vi "NVH_TEST.vi"(10 "振动2NHV-FFT":refnum<vi>, 11 "振动1NVH-FFT":refnum<vi>) -> ()   [LabVIEW 2020]
uses:
  Global_Variable/Global.vi
panel:
  out "error out":errorcluster caption="错误输出"
  in  "error in":errorcluster caption="错误输入"
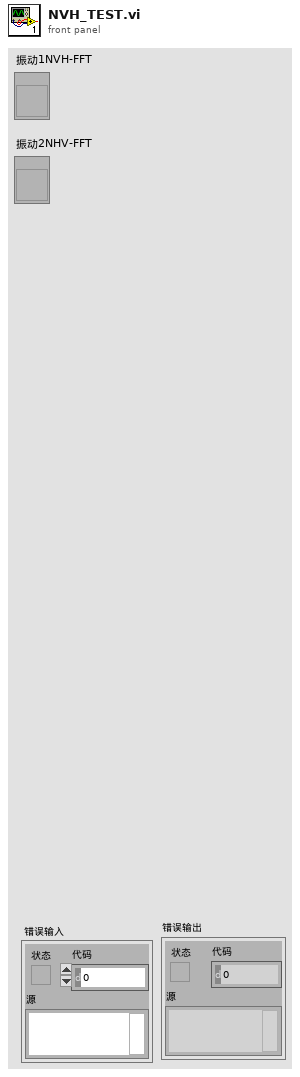
[diagram p1: front panel]
types:
  T1 = typedef "svc_Spectrum Info.ctl" = cluster{"channel name":string, "description":string, "x-axis units":T2, "spectral info":cluster{"spectrum type":T3, "linear/dB":enum16{"linear", "dB"}, "window":u16, "window size":i32, "FFT size":i32}, "engineering units":T4, "custom label":string, "dB reference [EU]":dbl, "peak units":enum16{"rms", "peak", "peak-peak"}, "weighting filter":T5, "spectral density?":bool, "unit label":string, "spectrum skewed?":bool, "complimentary spectrum units":T6}
  T2 = typedef "svc_X-Axis Units.ctl" = u16
  T3 = typedef "svc_Spectrum Type.ctl" = enum16{"FFT Spectrum [complex]", "Amplitude [Magnitude]", "Power [Magnitude^2]", "Cross Spectrum [complex]", "Frequency Response [Complex]"}
  T4 = typedef "svc_Engineering Units Text Ring.ctl" = u16
  T5 = typedef "svc_Weighting Filter Text Ring.ctl" = u16
  T6 = typedef "svc_Complimentary Spectrum Units.ctl" = enum16{"none", "radians", "degrees", "cycles", "imaginary"}
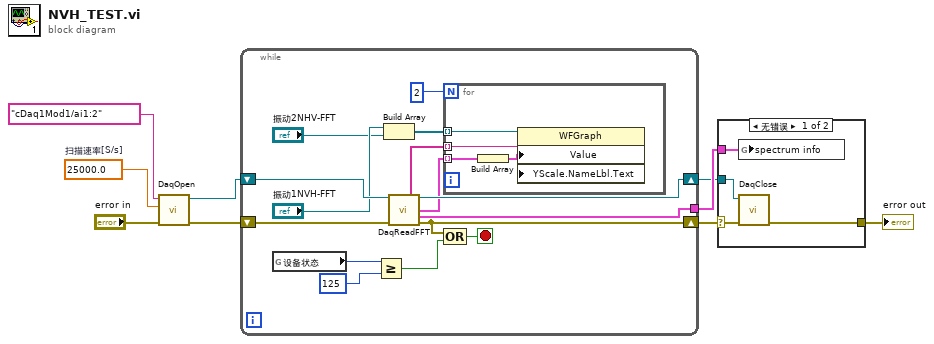
[diagram p0: block diagram]
diagram:
  w1 = 25000.0  # 扫描速率[S/s]
  n1 = call "DaqOpen.vi"("error in"="error in", "扫描速率[S/s]"=w1, "通道输入"=tag "cDaq1Mod1/ai1:2" ("DAQmx物理通道")) -> ("error out"=w9:errorcluster, "task out"=w3:refnum<k21>)  [unwired: 7 in]
  n2 = while {
    shift-right: [w23] -> w4
    shift-left: w3 -> [w24]
    shift-right: [w22] -> w5
    shift-left: w9 -> [w19]
    tunnel: [w20] -> w7
    stop <- w21 stop-if-true
    n3 = global read "Global.vi" "设备状态"() -> (w11:i16)
    n4 = Greater Or Equal?(x=w11, y=i16 125) -> (x >= y?=w12:bool)
    n5 = Build Array("振动1NVH-FFT", "振动2NHV-FFT") -> (w16:refnum<vi>[])
    n6 = call "DaqReadFFT.vi"("任务输入"=w24, "error in"=w19) -> ("unit labels"=w14:string[], "task out 2"=w23:refnum<k21>, "power spectra [dB EU]"=w15:cluster{"f0":dbl, "df":dbl, "magnitude":dbl[]}[], "spectrum info"=w20:T1[], "error out"=w22:errorcluster)  [unwired: 8 in, 1 out]
    n7 = for {
      N: 2 -> [_]
      tunnel: w16 -> [w28] mode=indexing
      tunnel: w15 -> [w27] mode=indexing
      tunnel: w14 -> [w26] mode=indexing
      n8 = Build Array(w27) -> (w25:cluster{"f0":dbl, "df":dbl, "magnitude":dbl[]}[])
      n9 = property class="WFGraph"(reference=w28, "Value"=w25, "YScale.NameLbl.Text"=w26) -> ()  [unwired: 1 in, 2 out]
    }
    n10 = Compound Arithmetic op=OR ("复合运算")(w22, w12) -> (w21:bool)
  }
  n11 = case shown="无错误" w5 {
    selector: w5 -> [w31 w33]
    tunnel: w4 -> [w32 _]
    tunnel: [w30 w33] -> w6
    tunnel: w7 -> [w29 _]
    frame No Error {
      n12 = global write "Global.vi" "spectrum info"(w29) -> ()
      n13 = call "DaqClose.vi"("error in"=w31, "task in"=w32) -> ("error out"=w30:errorcluster)  [unwired: 9 in]
    }
    frame Error {
    }
  }
  "error out" <- w6
